vi "Last Ack Created Queue.vi"(10 "Queue":refnum<class "Queue.lvclass">, 11 "TEMPLATE Queue in":refnum<class "TEMPLATE Queue.lvclass">) -> (3 "TEMPLATE Queue out":refnum<class "TEMPLATE Queue.lvclass">)   [LabVIEW 2021, in "_Template.lvlib" / "Templates.lvlib" / "TEMPLATE Queue.lvlib" / "TEMPLATE Queue.lvclass"]
uses:
  TEMPLATE Queue.lvclass
  <vilib>/Nathan Davis/jettl/jettl/Queue/Queue.lvclass
  TEMPLATE Queue.lvclass/TEMPLATE Queue.ctl
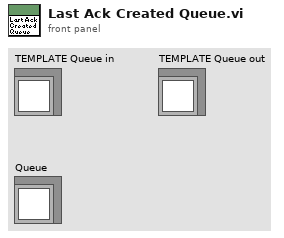
[diagram p1: front panel]
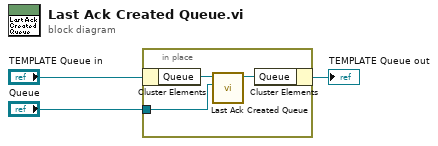
[diagram p0: block diagram]
diagram:
  n1 = in-place {
    in-place-border: "Queue" -> [w4]
    n2 = in-place-cluster #1("TEMPLATE Queue in") -> ("Queue"=w6:refnum<class "Queue.lvclass">)
    n3 = call-dynamic "Last Ack Created Queue.vi"("Queue"=w4, "jettl Msg Last Ack Created Queue in"=w6) -> ("jettl Msg Last Ack Created Queue out"=w5:refnum<class "Queue.lvclass">)  [unwired: 9 in]
    n4 = in-place-cluster #1("Queue"=w5) -> (→"TEMPLATE Queue out":refnum<class "TEMPLATE Queue.lvclass">)
  }
